vi "Prompt for Step--UI Interlocks.vi"(8 "error in (no error)":errorcluster, 10 "Control Refs":refnum<vi>[](array[refnum]), 11 "Window Action in":refnum<class "Window Action.lvclass">) -> (0 "error out":errorcluster, 2 "Step Valid?":bool, 3 "Window Action out":refnum<class "Window Action.lvclass">)   [LabVIEW 2020, in "MacroAssert.lvlib" / "Window Action.lvclass"]
uses:
  Window Action.lvclass
  Action Step/Action Step.lvclass
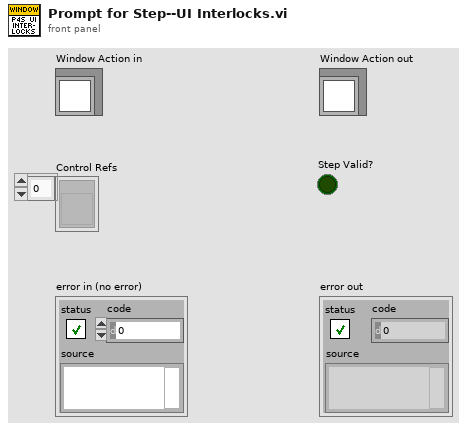
[diagram p1: front panel]
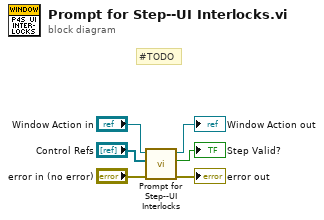
[diagram p0: block diagram]
diagram:
  # "#TODO"
  n1 = call-parent "Prompt for Step--UI Interlocks.vi"("error in (no error)"="error in (no error)", "Control Refs"="Control Refs", "Step in"="Window Action in") -> ("error out"=→"error out":errorcluster, "Step Valid?"=→"Step Valid?":bool, "Step out"=→"Window Action out":refnum<class "Window Action.lvclass">)  [unwired: 6 in]
